vi "XLP80_CAN_ErrorCodes.vi"() -> ()   [LabVIEW 2021]
panel:
  out "S91_SYS_Error_Code":u32[](array[numeric]) format="%.0x"
  out "ErrorMessage":string[](array[string])
  out "Array":string[](array[string])
  out "array":string[][](array[string])
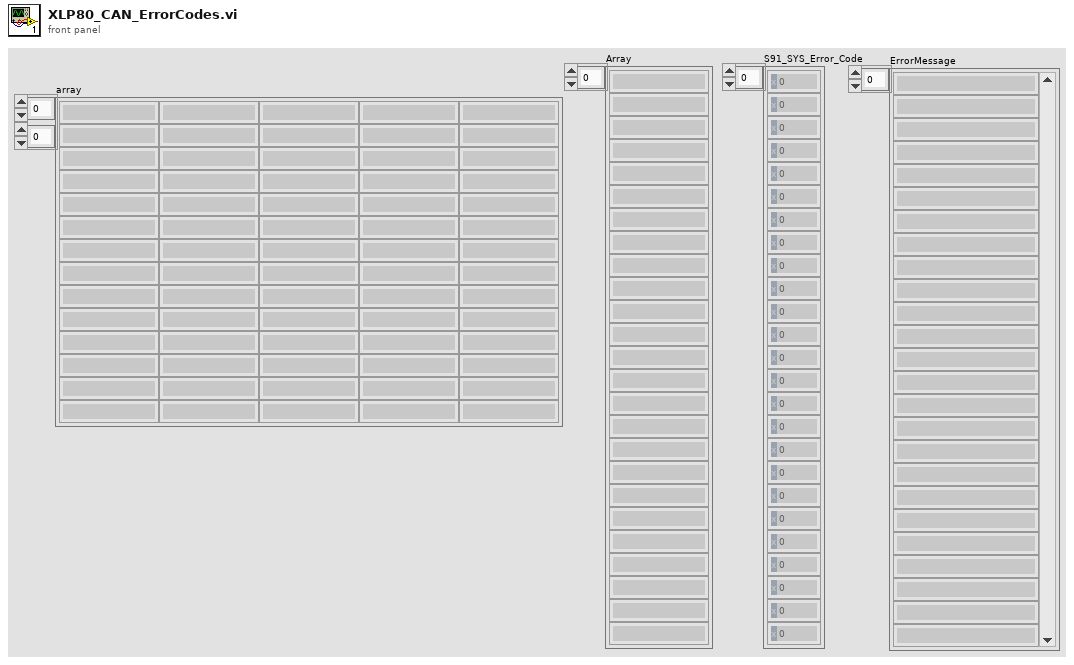
[diagram p1: front panel]
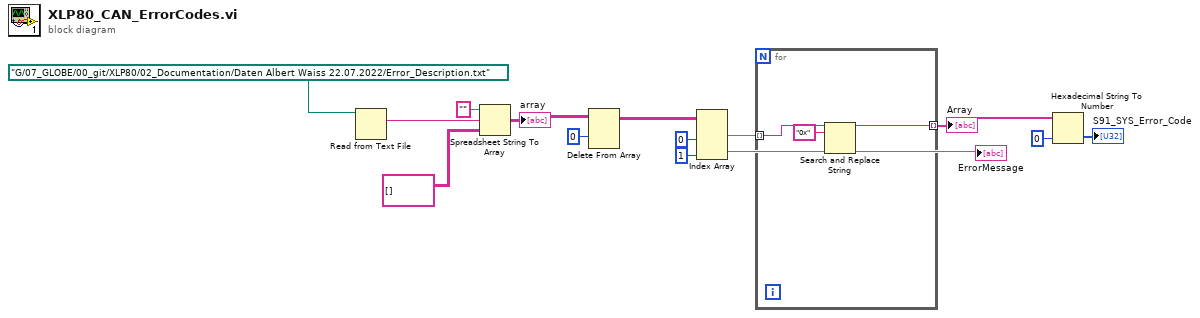
[diagram p0: block diagram]
diagram:
  n1 = Read from Text File(file (use dialog)=path "G:/07_GLOBE/00_git/XLP80/02_Documentation/Daten Albert Waiss 22.07.2022/Error_Description.txt") -> (text=w13:string)  [unwired: 3 in, 3 out]
  n2 = Spreadsheet String To Array(format string="", spreadsheet string=w13, array type (2D Dbl)=string[][] []) -> (array=w10:string[][])  [unwired: 1 in]
  "array" <- w10
  n3 = Delete From Array(array=w10, index (row)=0) -> (array with subset deleted=w8:string[][])  [unwired: 2 in, 1 out]
  n4 = Index Array(array=w8, index (col) #1=0 ("disabled index (col)"), index (col) #2=1 ("index (col)")) -> (element #1=w6:string[], element #2=→"ErrorMessage":string[])  [unwired: 2 in]
  n5 = for {
    tunnel: w6 -> [w17] mode=indexing
    tunnel: [w15] -> w3 mode=indexing
    n6 = Search and Replace String(input string=w17, search string="0x") -> (result string=w15:string)  [unwired: 6 in, 3 out]
  }
  "Array" <- w3
  n7 = Hexadecimal String To Number(string=w3, default (0uL)=u32 0 ("default (0 U32)")) -> (number=→"S91_SYS_Error_Code":u32[])  [unwired: 1 in, 1 out]
